vi "UART Stop.vi"(8 "Error In":errorcluster, 11 "FPGA VI Reference In":refnum<k20>) -> (0 "Error Out":errorcluster, 3 "FPGA VI Reference Out":refnum<k20>)   [LabVIEW 2018]
uses:
  <vilib>/FPGAPlugInAG/PXIe-5840/niLvFpga_Reset_PXIe-5840.vi
  <vilib>/rvi/interface/nirviMethod/nirviMethod.xnode
  Program Files (x86)/National Instruments/LabVIEW 2018/instr.lib/niVST/FPGA/Templates/FPGA Bitfiles/niVSTFPGA_UART.lvbitx
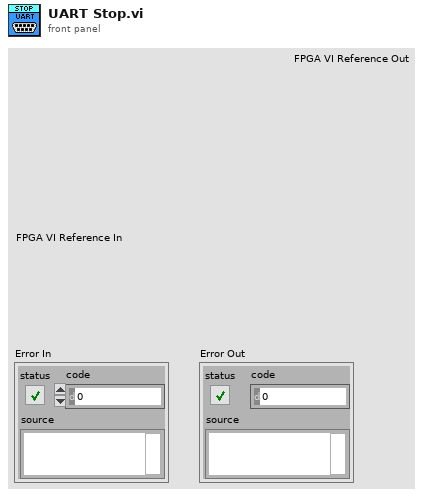
[diagram p1: front panel]
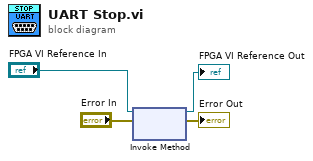
[diagram p0: block diagram]
diagram:
  n1 = xnode "Invoke Method"("FPGA VI Reference In"="FPGA VI Reference In", "error in"="Error In") -> ("FPGA VI Reference Out"=→"FPGA VI Reference Out":refnum<k20>, "error out"=→"Error Out":errorcluster)
